vi "UDP Server Digital Output.vi"(8 "error in (no error)":errorcluster, 10 "User Event in":refnum<class "User Event.lvclass">, 11 "UDP Port":u16=5005) -> (0 "error out":errorcluster)   [LabVIEW 2016]
uses:
  User Events/User Event.lvclass
  TypeDefs/DigitalOutput.ctl
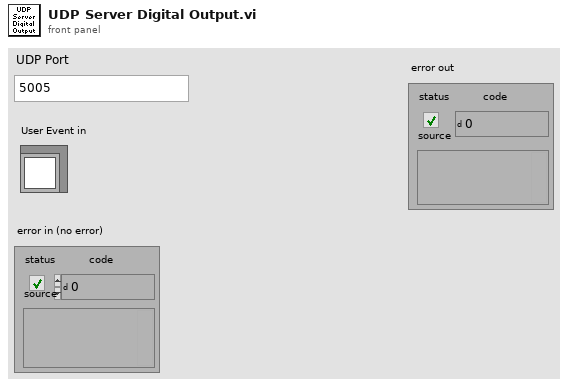
[diagram p1: front panel]
types:
  T1 = typedef "DigitalOutput.ctl" = cluster{"DigitalOutput":u8[], "Address":u32}
  T2 = typedef "M1M3SupSimUserEvents.ctl" = cluster{"ILCResponse":refnum<user-event>, "StopUDPServer":refnum<user-event>, "InclinometerResponse":refnum<user-event>, "DisplaceResponse":refnum<user-event>, "AccelerometerResponse":refnum<user-event>, "DigitalInput":refnum<user-event>, "DigitalOutput":refnum<user-event>, "GyroResponse":refnum<user-event>}
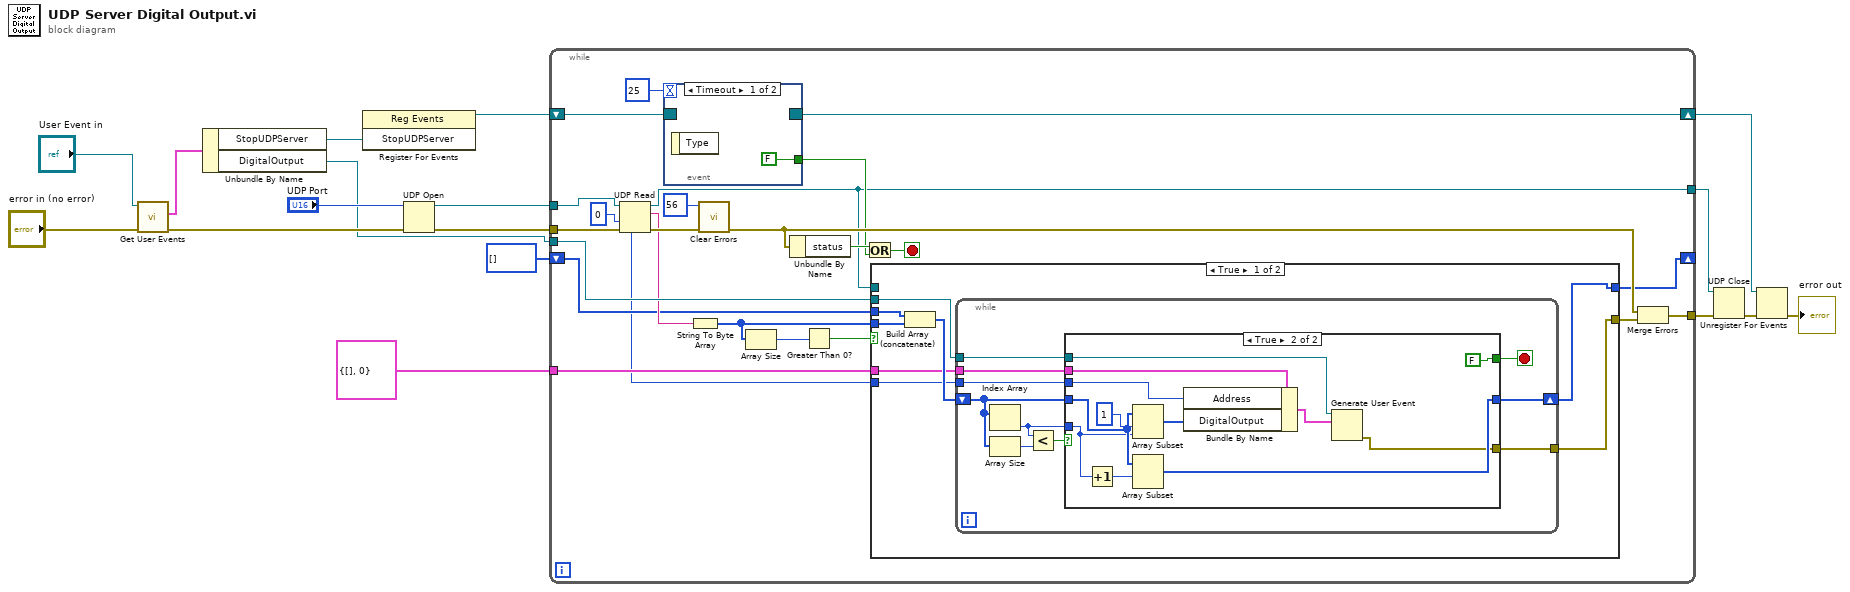
[diagram p0: block diagram]
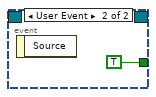
[diagram p2: hidden frame]
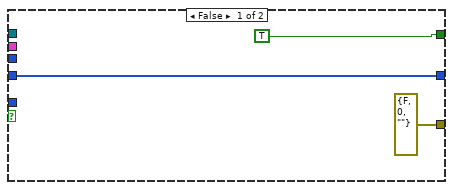
[diagram p3: hidden frame]
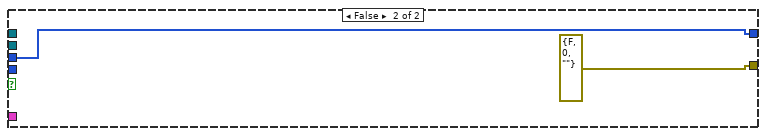
[diagram p4: hidden frame]
diagram:
  n1 = call "Get User Events.vi"("error in (no error)"="error in (no error)", "User Event in"="User Event in") -> ("error out"=w17:errorcluster, "User Events"=w14:T2)  [unwired: 7 in, 1 out]
  n2 = Unbundle By Name(w14) -> ("StopUDPServer"=w15:refnum<user-event>, "DigitalOutput"=w2:refnum<user-event>)
  n3 = register-events(w15) -> (reference out=w9:refnum<event-registration>)  [unwired: 2 in, 1 out]
  n4 = UDP Open(8:w17, 11:"UDP Port") -> (port=w5:refnum<k16>, 0:w6:errorcluster)  [unwired: 3 in, 1 out]
  n5 = while {
    tunnel: w5 -> [w41]
    tunnel: w6 -> [w40]
    tunnel: [w33] -> w8
    tunnel: [w26] -> w7
    shift-right: [w28] -> w11
    shift-left: w9 -> [w31]
    tunnel: w2 -> [w27]
    shift-right: [w23] -> _
    shift-left: u8[] [] ("unsigned byte array") -> [w24]
    tunnel: T1 {"DigitalOutput"=[], "Address"=0} ("DigitalOutputCluster") -> [w19]
    stop <- w32 stop-if-true
    n6 = UDP Read(connection ID=w41, timeout ms (25000)=0, 8:w40) -> (data out=w25:string, error out=w38:errorcluster, 3:w26:refnum<k16>, 6:w18:u32)  [unwired: 1 in, 1 out]
    n7 = event shown="[0] Timeout" {
      selector: w31 -> [_ _]
      dyn-events: [_ _] -> w28
      timeout: 25 -> [_ _]
      tunnel: [FALSE TRUE] -> w29
      event Timeout {
        n8 = event-data() -> ()  [unwired: 1 in, 1 out]
      }
      event User Event {
        n9 = event-data() -> ()  [unwired: 1 in, 1 out]
      }
    }
    n10 = String To Byte Array(string=w25) -> (unsigned byte array=w22:u8[])
    n11 = call <vilib>:"Clear Errors.vi"("error in (no error)"=w38, "specific error code to clear (0: all)"=56) -> ("error out"=w35:errorcluster)  [unwired: 4 in, 1 out]
    n12 = Array Size(array=w22) -> (size(s)=w21:i32)
    n13 = Unbundle By Name(w35) -> ("status"=w36:bool)
    n14 = Greater Than 0?(x=w21) -> (x > 0?=w20:bool)
    n15 = Or(x=w36, y=w29) -> (x .or. y?=w32:bool)
    n16 = case shown="True" w20 {
      tunnel: [w44 errorcluster {"status"=FALSE, "code"=0, "source"=""} ("error out")] -> w34
      tunnel: w27 -> [w48 _]
      tunnel: w26 -> [_ _]
      tunnel: w22 -> [w50 _]
      tunnel: w24 -> [w51 w77]
      tunnel: [w47 w77] -> w23
      tunnel: w19 -> [w46 _]
      tunnel: w18 -> [w45 _]
      frame True {
        n17 = Build Array (concatenate)(w51, w50) -> (w49:u8[])
        n18 = while {
          tunnel: w48 -> [w60]
          shift-right: [w58] -> w47
          shift-left: w49 -> [w57]
          tunnel: w46 -> [w54]
          tunnel: w45 -> [w53]
          tunnel: [w52] -> w44
          stop <- w59 stop-if-true
          n19 = Index Array(array=w57) -> (element=w55:u8)  [unwired: 1 in]
          n20 = Array Size(array=w57) -> (size(s)=w56:i32)
          n21 = Less?(x=w55, y=w56) -> (x < y?=w61:bool)
          n22 = case shown="True" w61 {
            tunnel: w57 -> [w64 w75]
            tunnel: w55 -> [_ w70]
            tunnel: w60 -> [_ w76]
            tunnel: [w64 w74] -> w58
            tunnel: [TRUE FALSE] -> w59
            tunnel: w54 -> [_ w69]
            tunnel: w53 -> [_ w67]
            tunnel: [errorcluster {"status"=FALSE, "code"=0, "source"=""} ("error out") w65] -> w52
            frame False {
            }
            frame True {
              n23 = Increment(x=w70) -> (x+1=w71:u8)
              n24 = Array Subset(array=w75, index=1, length=w70) -> (w68:u8[])
              n25 = Array Subset(array=w75, index=w71) -> (w74:u8[])  [unwired: 1 in]
              n26 = Bundle By Name(cluster=w69, "Address"=w67, "DigitalOutput"=w68) -> (w66:T1)
              n27 = Generate User Event(user event=w76, event data cluster=w66) -> (error out=w65:errorcluster)  [unwired: 2 in, 1 out]
            }
          }
        }
      }
      frame False {
      }
    }
    n28 = Merge Errors(w35, w34) -> (w33:errorcluster)
  }
  n29 = UDP Close(connection ID=w7, 8:w8) -> (error out=w10:errorcluster)  [unwired: 1 out]
  n30 = Unregister For Events(event registration refnum=w11, error in=w10) -> (error out=→"error out":errorcluster)
